vi "Raw_Table_SubarraySel.vi"(2 "error in (no error)":errorcluster, 3 "Column Index":i32, 4 "String to compare":string, 5 "Raw Bar Table Data":string[][](array[string])) -> (0 "error out":errorcluster, 1 "Output":string[][](array[string]))   [LabVIEW 2017]
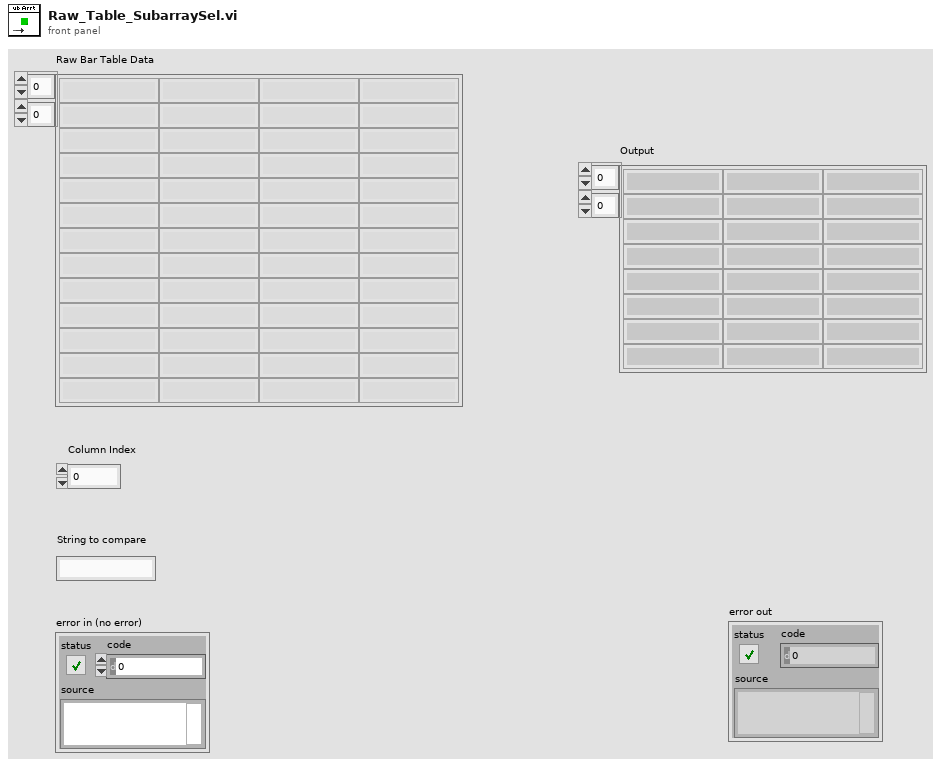
[diagram p1: front panel]
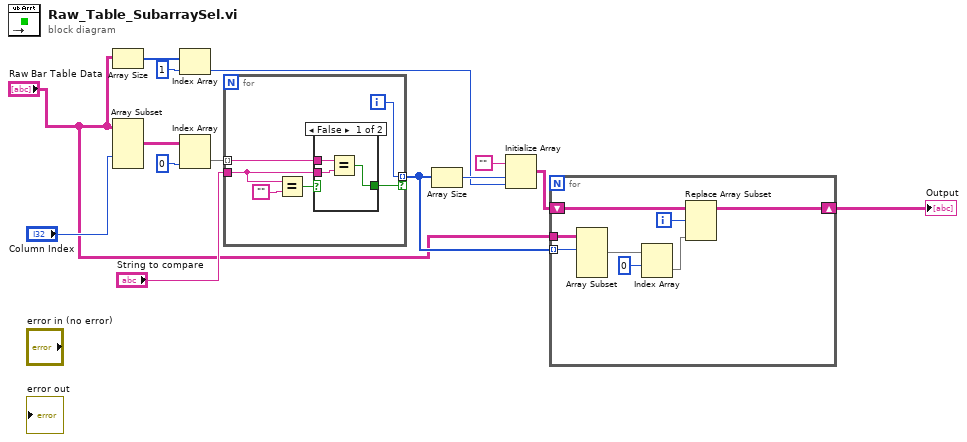
[diagram p0: block diagram]
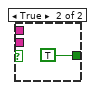
[diagram p2: hidden frame]
diagram:
  n1 = Array Size(array="Raw Bar Table Data") -> (size(s)=w8:i32[])
  n2 = Array Subset(array="Raw Bar Table Data", index (col)="Column Index") -> (w3:string[][])  [unwired: 3 in]
  n3 = Index Array(array=w8, index=1) -> (element=w6:i32)
  n4 = Index Array(array=w3, index (col)=0 ("disabled index (col)")) -> (element=w9:string[])  [unwired: 1 in]
  n5 = for {
    tunnel: w9 -> [w17] mode=indexing
    tunnel: "String to compare" -> [w15]
    tunnel: [w20] -> w11 mode=indexing if=w16
    i -> [w20]
    n6 = Equal?(x=w15, y="") -> (x = y?=w19:bool)
    n7 = case shown="False" w19 {
      tunnel: w17 -> [w23 _]
      tunnel: [w21 TRUE] -> w16
      tunnel: w15 -> [w22 _]
      frame False {
        n8 = Equal?(x=w23, y=w22) -> (x = y?=w21:bool)
      }
      frame True {
      }
    }
  }
  n9 = Array Size(array=w11) -> (size(s)=w10:i32)
  n10 = Initialize Array("", w10, w6) -> (w5:string[][])
  n11 = for {
    tunnel: "Raw Bar Table Data" -> [w32]
    tunnel: w11 -> [w31] mode=indexing
    shift-right: [w28] -> w2
    shift-left: w5 -> [w29]
    i -> [w30]
    n12 = Array Subset(array=w32, index (row)=w31) -> (w27:string[][])  [unwired: 3 in]
    n13 = Index Array(array=w27, index (row)=0) -> (element=w25:string[])  [unwired: 1 in]
    n14 = Replace Array Subset(array=w29, new element=w25, index (row)=w30) -> (w28:string[][])  [unwired: 1 in]
  }
  "Output" <- w2
